vi "Main.vi"(11 "Module Admin":refnum<class "Delacor_lib_QMH_Module Admin.lvclass">) -> ()   [LabVIEW 2019, in "Rotation Stage.lvlib"]
doc: "This template is based off of the Queued Message Handler design pattern and the Queued Message Handler project template that ships with LabVIEW.\n\nThe main difference is that the queue is private to this module and communication between modules is performed via Broadcast and Request events.\n\nRequest events are wrapped in public API methods and are handled in the Event Handling Loop (EHL) of this VI. Any module can register for Broadcast events sent by this module. The EHL generates messages based on user interface actions.\n\nThe Message Handling Loop (MHL) processes messages generated by the EHL, or by other messages. The messages are string values, so new messages can be added easily to the Message Cases case structure in the MHL. Each message cluster can also provide an optional value for Message Data, which is a variant that can be converted to whatever message-specific data is required.\n_____\nBased on Delacor QMH Project Template 5.0.0.82."
uses:
  Rotation Stage.lvlib
  <vilib>/Delacor/Delacor QMH/Libraries/Module Admin_class/Delacor_lib_QMH_Module Admin.lvclass
  Module Data--cluster.ctl
  Stop Argument--cluster.ctl
  <vilib>/Delacor/Delacor QMH/Libraries/Message Queue_class/Delacor_lib_QMH_Message Queue.lvclass/Delacor_lib_QMH_Message Queue.ctl
  <vilib>/Delacor/Delacor QMH/Libraries/Module Admin_class/Delacor_lib_QMH_Module Admin.lvclass/Delacor_lib_QMH_Module Admin.ctl
  Get Position Argument--cluster.ctl
  Get Position (Reply Payload)--cluster.ctl
  Set Position Argument--cluster.ctl
  Get Module Data Argument--cluster.ctl
  Get Module Data (Reply Payload)--cluster.ctl
  <vilib>/Utility/miscctls.llb/LVPointTypeDef.ctl
  <vilib>/Delacor/Delacor QMH/Libraries/Message Queue_class/Delacor_lib_QMH_Enqueue Message (Single).vi
  <vilib>/Delacor/Delacor QMH/Libraries/Module Admin_class/Delacor_lib_QMH_Get External Launch.vi
  <vilib>/Utility/error.llb/Error Cluster From Error Code.vi
  <vilib>/ErrorRing/Error Ring.xnode
  <vilib>/Delacor/Delacor QMH/Libraries/Message Queue_class/Delacor_lib_QMH_Message Queue.lvclass
panel:
  in  "MG17Motor":refnum<k7>(container)
  out "error out":errorcluster
  out "Status":string
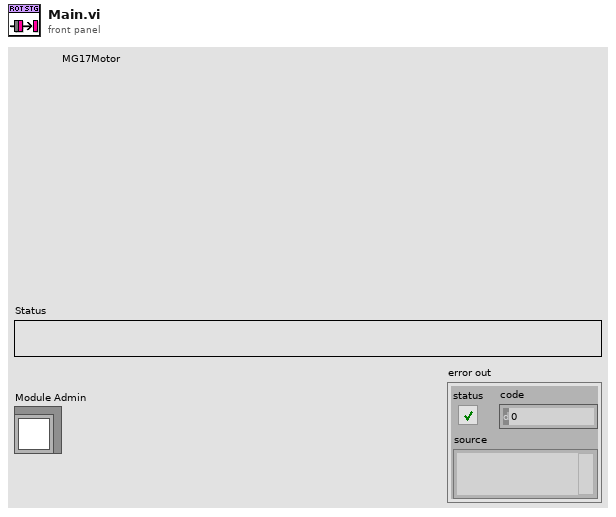
[diagram p1: front panel]
types:
  T1 = typedef "Rotation Stage.lvlib/Request Events--cluster.ctl" = cluster{"Stop Module":refnum<user-event>, "Show Panel":refnum<user-event>, "Hide Panel":refnum<user-event>, "Get Module Execution Status":refnum<user-event>, "Show Diagram":refnum<user-event>, "Get Position":refnum<user-event>, "Set Position":refnum<user-event>, "Get Module Data":refnum<user-event>}
  T2 = typedef "Rotation Stage.lvlib/Module Data--cluster.ctl" = cluster{"-Status":string, "-Reference":refnum<k7>, "Position":sgl}
  T3 = enum32{"invalid lock state", "Not Locked", "Locked (No Password)", "Password-protected"}
  T4 = typedef "Rotation Stage.lvlib/Stop Argument--cluster.ctl" = cluster{"Origin":string, "Exit via Stop Module Req?":bool, "Wait for Module to stop?":bool}
  T5 = typedef "Rotation Stage.lvlib/Get Position Argument--cluster.ctl" = cluster{"Wait Notifier":refnum<notifier>, "wait for reply":bool}
  T6 = typedef "Rotation Stage.lvlib/Set Position Argument--cluster.ctl" = cluster{"Position":sgl, "Wait":bool}
  T7 = typedef "Rotation Stage.lvlib/Get Module Data Argument--cluster.ctl" = cluster{"Wait Notifier":refnum<notifier>, "wait for reply":bool}
  T8 = typedef "LVPointTypeDef.ctl" = cluster{"Horizontal":i16, "Vertical":i16}
  T9 = enum32{"Invalid", "Standard", "Closed", "Hidden", "Minimized", "Maximized"}
  T10 = typedef "Rotation Stage.lvlib/Get Position (Reply Payload)--cluster.ctl" = cluster{"Position":dbl, "Get Position_error":errorcluster}
  T11 = typedef "Rotation Stage.lvlib/Get Module Data (Reply Payload)--cluster.ctl" = cluster{"Rotation Stage":T2, "Get Module Data_error":errorcluster}
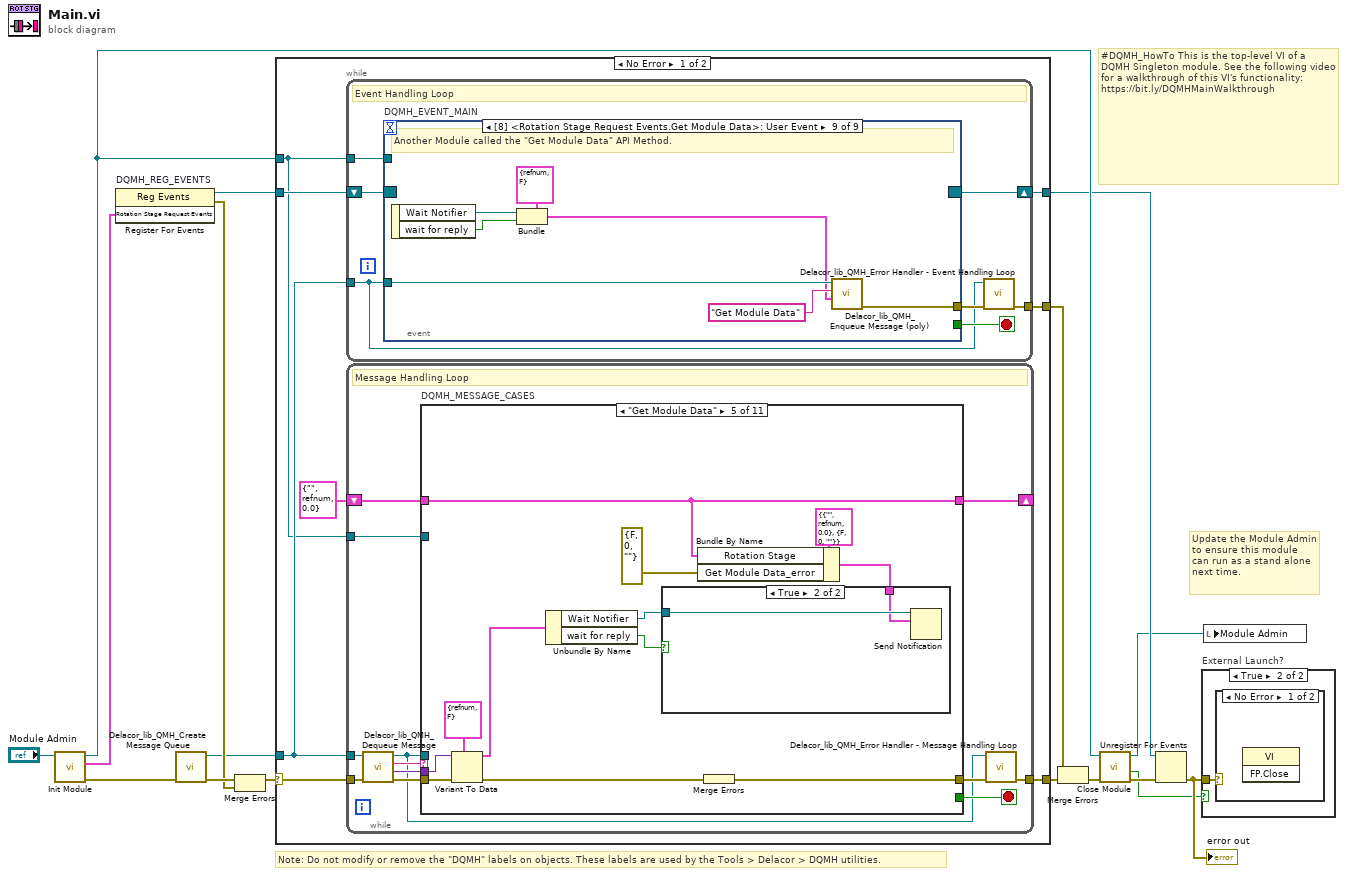
[diagram p0: block diagram]
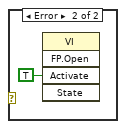
[diagram p3: hidden frame]
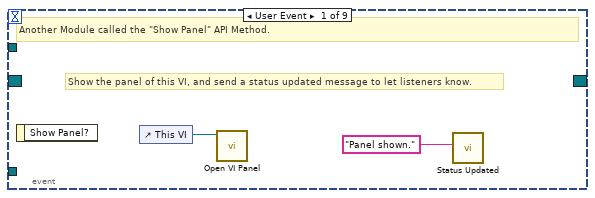
[diagram p4: hidden frame]
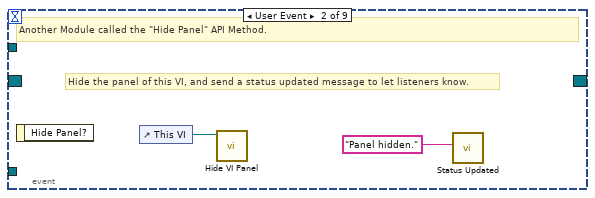
[diagram p5: hidden frame]
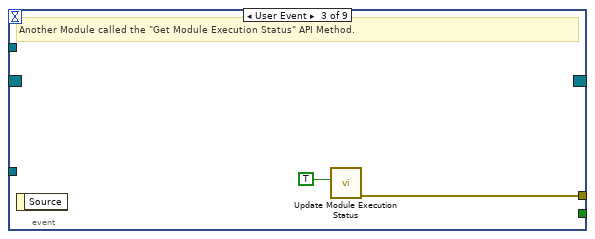
[diagram p6: hidden frame]
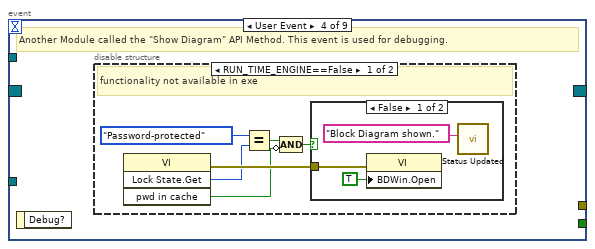
[diagram p7: hidden frame]
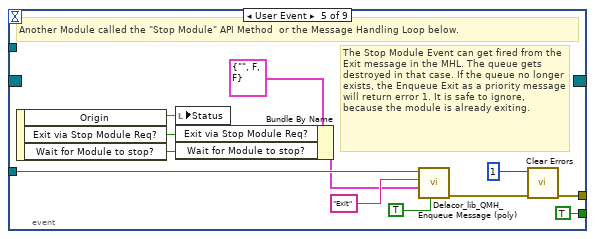
[diagram p10: hidden frame]
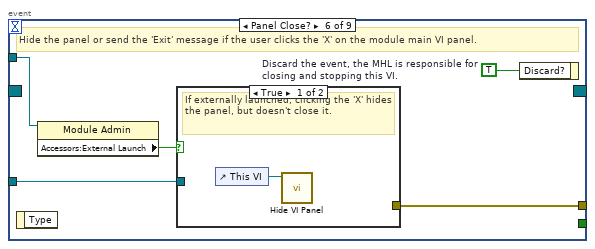
[diagram p11: hidden frame]
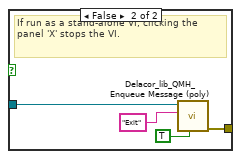
[diagram p12: hidden frame]
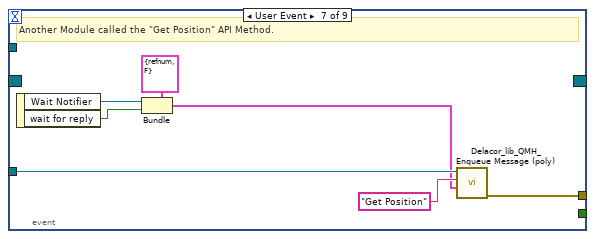
[diagram p13: hidden frame]
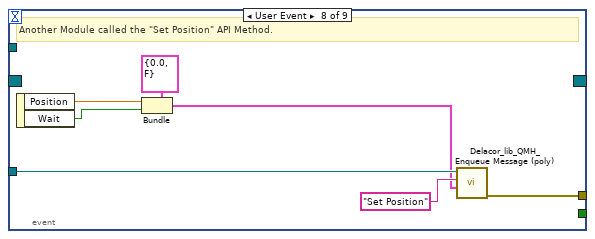
[diagram p14: hidden frame]
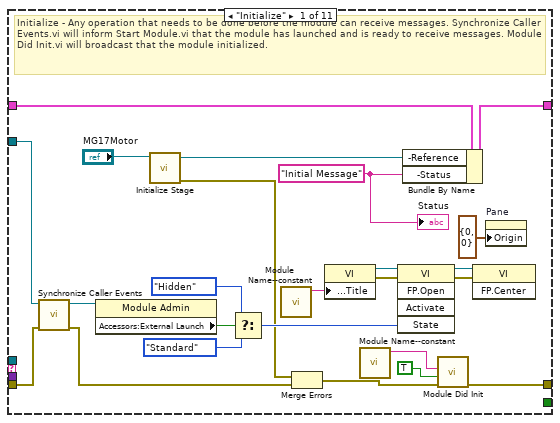
[diagram p15: hidden frame]
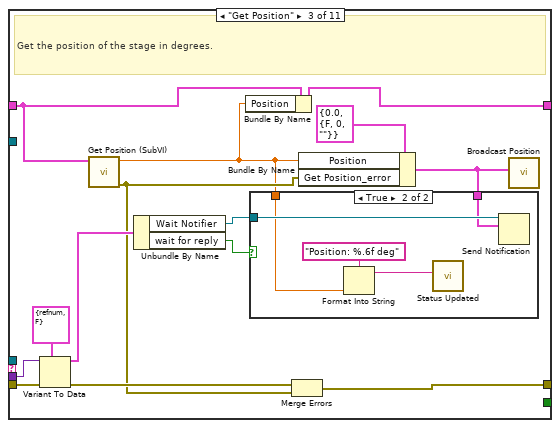
[diagram p17: hidden frame]
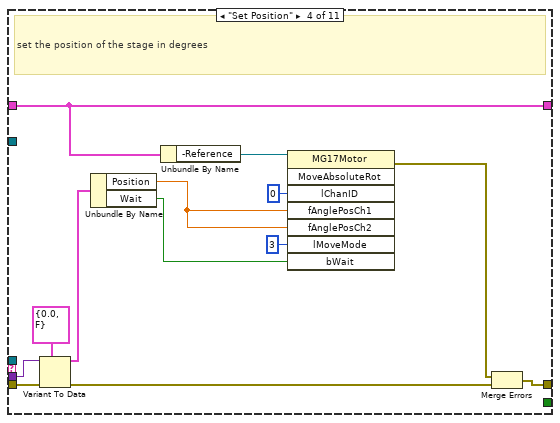
[diagram p19: hidden frame]
diagram:
  # "#DQMH_HowTo This is the top-level VI of a DQMH Singleton module. See the following video for a walkthrough of this VI's functionality: https://bit.ly/DQMHMainWalkthrough"
  # "Note: Do not modify or remove the \"DQMH\" labels on objects. These labels are used by the Tools > Delacor > DQMH utilities."
  # "Update the Module Admin to ensure this module can run as a stand alone next time."
  n1 = call "Init Module.vi"("Singleton Module Admin in"="Module Admin") -> ("error out"=w16:errorcluster, "Rotation Stage Request Events"=w5:T1, "Singleton Module Admin out"=w8:refnum<class "Delacor_lib_QMH_Module Admin.lvclass">)  [unwired: 8 in]
  n2 = register-events "DQMH_REG_EVENTS"(w5) -> (reference out=w6:refnum<event-registration>, error out=w9:errorcluster)  [unwired: 2 in]
  n3 = call <vilib>:"Delacor_lib_QMH_Create Message Queue.vi"("error in (no error)"=w16) -> ("error out"=w11:errorcluster, "Message Queue"=w4:refnum<class "Delacor_lib_QMH_Message Queue.lvclass">)  [unwired: 9 in]
  n4 = Merge Errors(w11, w9) -> (w10:errorcluster)
  n5 = case shown="No Error" w10 {
    selector: w10 -> [w23 w240]
    tunnel: [w25 w239] -> w17
    tunnel: [w22 w245] -> w7
    tunnel: w6 -> [w20 w245]
    tunnel: w4 -> [w19 w238]
    tunnel: [w24 _] -> w14
    tunnel: w8 -> [w18 w241]
    frame No Error {
      n6 = while {
        tunnel: w19 -> [w26]
        shift-right: [w29] -> w22
        shift-left: w20 -> [w30]
        tunnel: [w31] -> w24
        tunnel: w18 -> [w27]
        stop <- w28 stop-if-true
        # "Event Handling Loop"
        n7 = event "DQMH_EVENT_MAIN" shown="[8] <Rotation Stage Request Events.Get Module Data>: User Event" {
          selector: w30 -> [_ _ _ _ _ _ _ _ _]
          dyn-events: [_ _ _ _ _ _ _ _ _] -> w29
          timeout: _ -> [_ _ _ _ _ _ _ _ _]
          tunnel: [_ _ _ _ TRUE ("Discard?") _ _ _ _] -> w28
          tunnel: w26 -> [_ _ _ _ w55 w62 w76 w83 w90]
          tunnel: [_ _ w38 _ w58 w64 w70 w78 w84] -> w32
          tunnel: w27 -> [_ _ _ _ _ w61 _ _ _]
          event User Event {
            # "Show the panel of this VI, and send a status updated message to let listeners know."
            # "Another Module called the \"Show Panel\" API Method."
            n8 = event-data() -> ()  [unwired: 1 in, 1 out]
            n9 = control-ref of="This VI"() -> (w34:refnum<vi>)
            n10 = call "Open VI Panel.vi"("VI"=w34) -> ()  [unwired: 10 in, 1 out]
            n11 = call "Status Updated.vi"("Status"="Panel shown." ("format string")) -> ()  [unwired: 10 in, 1 out]
          }
          event User Event {
            # "Hide the panel of this VI, and send a status updated message to let listeners know."
            # "Another Module called the \"Hide Panel\" API Method."
            n12 = event-data() -> ()  [unwired: 1 in, 1 out]
            n13 = control-ref of="This VI"() -> (w36:refnum<vi>)
            n14 = call "Hide VI Panel.vi"("VI"=w36) -> ()  [unwired: 10 in, 1 out]
            n15 = call "Status Updated.vi"("Status"="Panel hidden." ("format string")) -> ()  [unwired: 10 in, 1 out]
          }
          event User Event {
            # "Another Module called the \"Get Module Execution Status\" API Method."
            n16 = event-data() -> ()  [unwired: 1 in, 1 out]
            n17 = call "Update Module Execution Status.vi"("Running?"=TRUE) -> ("error out"=w38:errorcluster)  [unwired: 10 in]
          }
          event User Event {
            # "Another Module called the \"Show Diagram\" API Method. This event is used for debugging."
            n18 = event-data() -> ()  [unwired: 1 in, 1 out]
            n19 = disable-structure shown="RUN_TIME_ENGINE==False" {
              frame condition #0 (active) {
                # "functionality not available in exe"
                n20 = invoke class="VI" method="Lock State.Get"() -> (error out=w44:errorcluster, "Get Lock State"=w43:T3, "pwd in cache"=w40:bool)  [unwired: 4 in, 1 out]
                n21 = Equal?(x=T3."Password-protected", y=w43) -> (x = y?=w41:bool)
                n22 = Compound Arithmetic op=AND(w41, invert w40) -> (w39:bool)
                n23 = case shown="False" w39 {
                  tunnel: w44 -> [w47 _]
                  frame False {
                    n24 = property class="VI"(error in=w47, "BDWin.Open"=TRUE ("Block Diagram Window:Open")) -> ()  [unwired: 1 in, 2 out]
                    n25 = call "Status Updated.vi"("Status"="Block Diagram shown." ("format string")) -> ()  [unwired: 10 in, 1 out]
                  }
                  frame True {
                    # "Password-protected VI, and the password is not in the cache. Do not show the diagram."
                  }
                }
              }
              frame condition #1 {
              }
            }
          }
          event User Event {
            # "The Stop Module Event can get fired from the Exit message in the MHL. The queue gets destroyed in that case. If the queue no longer exists, the Enqueue Exit as a priority message will return error 1. It is safe to ignore, because the module is already exiting."
            # "Another Module called the \"Stop Module\" API Method  or the Message Handling Loop below."
            n26 = event-data() -> ("Origin"=w54:string, "Exit via Stop Module Req?"=w50:bool, "Wait for Module to stop?"=w49:bool)  [unwired: 1 in]
            n27 = local write "Status"(w54) -> ()
            n28 = Bundle By Name(cluster=T4 {"Origin"="", "Exit via Stop Module Req?"=FALSE, "Wait for Module to stop?"=FALSE} ("Stop Argument"), "Exit via Stop Module Req?"=w50, "Wait for Module to stop?"=w49) -> (w48:T4)
            n29 = call-poly <vilib>:"Delacor_lib_QMH_Enqueue Message (poly).vi"("Priority Message? (F)"=TRUE, "Message Data"=w48, "Message"="Exit", "Message Queue in"=w55) -> ("error out"=w59:errorcluster)  [unwired: 6 in, 1 out]
            n30 = call <vilib>:"Clear Errors.vi"("error in (no error)"=w59, "specific error code to clear (0: all)"=1) -> ("error out"=w58:errorcluster)  [unwired: 4 in, 1 out]
          }
          event Panel Close? {
            w63 = TRUE  # Discard the event, the MHL is responsible for closing and stopping this VI.
            # "Hide the panel or send the 'Exit' message if the user clicks the 'X' on the module main VI panel."
            n31 = event-data() -> ()  [unwired: 1 in, 1 out]
            n32 = property class="Module Admin"(reference=w61) -> ("Accessors:External Launch"=w60:bool)  [unwired: 1 in, 2 out]
            n33 = case shown="True" w60 {
              tunnel: w62 -> [_ w68]
              tunnel: [_ w69] -> w64
              frame True {
                # "If externally launched, clicking the 'X' hides the panel, but doesn't close it."
                n34 = control-ref of="This VI"() -> (w65:refnum<vi>)
                n35 = call "Hide VI Panel.vi"("VI"=w65) -> ()  [unwired: 10 in, 1 out]
              }
              frame False {
                # "If run as a stand-alone VI, clicking the panel 'X' stops the VI."
                n36 = call-poly <vilib>:"Delacor_lib_QMH_Enqueue Message (poly).vi"("Priority Message? (F)"=TRUE, "Message"="Exit", "Message Queue in"=w68) -> ("error out"=w69:errorcluster)  [unwired: 7 in, 1 out]
              }
            }
            n37 = event-data("Discard?"=w63) -> ()  [unwired: 1 in, 1 out]
          }
          event User Event {
            # "Another Module called the \"Get Position\" API Method."
            n38 = event-data() -> ("Wait Notifier"=w72:refnum<notifier>, "wait for reply"=w71:bool)  [unwired: 1 in]
            n39 = Bundle(cluster=T5 {"Wait Notifier"=refnum, "wait for reply"=FALSE} ("Get Position Argument"), "Wait Notifier"=w72, "wait for reply"=w71) -> (w73:T5)
            n40 = call-poly <vilib>:"Delacor_lib_QMH_Enqueue Message (poly).vi"("Message Data"=w73, "Message"="Get Position", "Message Queue in"=w76) -> ("error out"=w70:errorcluster)  [unwired: 7 in, 1 out]
          }
          event User Event {
            # "Another Module called the \"Set Position\" API Method."
            n41 = event-data() -> ("Position"=w79:sgl, "Wait"=w77:bool)  [unwired: 1 in]
            n42 = Bundle(cluster=T6 {"Position"=0.0, "Wait"=FALSE} ("Set Position Argument"), "Position"=w79, "Wait"=w77) -> (w80:T6)
            n43 = call-poly <vilib>:"Delacor_lib_QMH_Enqueue Message (poly).vi"("Message Data"=w80, "Message"="Set Position", "Message Queue in"=w83) -> ("error out"=w78:errorcluster)  [unwired: 7 in, 1 out]
          }
          event User Event {
            # "Another Module called the \"Get Module Data\" API Method."
            n44 = event-data() -> ("Wait Notifier"=w86:refnum<notifier>, "wait for reply"=w85:bool)  [unwired: 1 in]
            n45 = Bundle(cluster=T7 {"Wait Notifier"=refnum, "wait for reply"=FALSE} ("Get Module Data Argument"), "Wait Notifier"=w86, "wait for reply"=w85) -> (w87:T7)
            n46 = call-poly <vilib>:"Delacor_lib_QMH_Enqueue Message (poly).vi"("Message Data"=w87, "Message"="Get Module Data", "Message Queue in"=w90) -> ("error out"=w84:errorcluster)  [unwired: 7 in, 1 out]
          }
        }
        n47 = call-dynamic "Delacor_lib_QMH_Error Handler - Event Handling Loop.vi"("error in (no error)"=w32, "Message Queue in"=w26) -> ("dup error in"=w31:errorcluster)  [unwired: 8 in, 1 out]
      }
      n48 = while {
        tunnel: w19 -> [w93]
        shift-right: [w97] -> _
        shift-left: T2 {"-Status"="", "-Reference"=refnum, "Position"=0.0} ("Data Cluster") -> [w98]
        tunnel: w23 -> [w101]
        tunnel: [w99] -> w25
        tunnel: w18 -> [w91]
        stop <- w96 stop-if-true
        # "Message Handling Loop"
        n49 = call-dynamic "Delacor_lib_QMH_Dequeue Message.vi"("error in (no error)"=w101, "Message Queue in"=w93) -> ("error out"=w100:errorcluster, "Message Data"=w94:variant, "Message"=w95:string, "Message Queue out"=w92:refnum<class "Delacor_lib_QMH_Message Queue.lvclass">)  [unwired: 6 in]
        n50 = case "DQMH_MESSAGE_CASES" shown="\"Get Module Data\"" w95 {
          selector: w95 -> [_ _ _ _ _ _ _ _ _ _ w225]
          tunnel: w92 -> [_ _ _ _ _ _ _ _ w195 w217 _]
          tunnel: w100 -> [w124 w128 w142 w160 w172 w177 w179 w184 w202 w223 w227]
          tunnel: [w122 w128 w133 w151 w163 w176 w179 w183 w198 w220 w228] -> w102
          tunnel: w98 -> [w113 w127 w132 w155 w162 w175 w178 w181 w197 w209 w226]
          tunnel: [w112 w127 w130 w155 w162 w175 w178 w181 w197 w209 w226] -> w97
          tunnel: [_ _ _ _ _ _ _ _ _ w216 _] -> w96
          tunnel: w94 -> [_ _ w140 w158 w170 _ _ _ w196 w215 _]
          tunnel: w91 -> [w114 _ _ _ _ _ _ _ w194 w210 _]
          frame "Initialize" {
            w107 = "Initial Message" ("Initial Message")
            # "Initialize - Any operation that needs to be done before the module can receive messages. Synchronize Caller Events.vi will inform Start Module.vi that the module has launched and is ready to receive messages. Module Did Init.vi will broadcast that the module initialized."
            n51 = call "Synchronize Caller Events.vi"("error in (no error)"=w124, "Singleton Module Admin in"=w114) -> ("error out"=w123:errorcluster, "Singleton Module Admin out"=w109:refnum<class "Delacor_lib_QMH_Module Admin.lvclass">)  [unwired: 8 in]
            n52 = property class="Module Admin"(reference=w109) -> ("Accessors:External Launch"=w118:bool)  [unwired: 1 in, 2 out]
            n53 = call "Initialize Stage.vi"("Automation Refnum in"="MG17Motor") -> ("error out"=w103:errorcluster, "reference out"=w105:refnum<k7>)  [unwired: 9 in]
            n54 = Select(t=T9."Hidden" ("State"), s=w118, f=T9."Standard" ("State")) -> (s? t:f=w115:T9)
            n55 = call "Module Name--constant.vi"() -> ("Module Name"=w121:string)  [unwired: 11 in]
            n56 = Merge Errors(w103, w123) -> (w104:errorcluster)
            n57 = property class="VI"("Front Panel.Title"=w121) -> (reference out=w120:refnum<vi>, error out=w126:errorcluster)  [unwired: 2 in]
            n58 = call "Module Name--constant.vi"() -> ("Module Name"=w110:string)  [unwired: 11 in]
            n59 = invoke class="VI" method="FP.Open"(reference=w120, error in=w126, "State"=w115) -> (reference out=w119:refnum<vi>, error out=w125:errorcluster)  [unwired: 2 in, 3 out]
            n60 = Bundle By Name(cluster=w113, "-Reference"=w105, "-Status"=w107) -> (w112:T2)
            n61 = call "Module Did Init.vi"("error in (no error)"=w104, "Initialized?"=TRUE, "Origin"=w110) -> ("error out"=w122:errorcluster)  [unwired: 8 in]
            n62 = invoke class="VI" method="FP.Center"(reference=w119, error in=w125) -> ()  [unwired: 1 in, 3 out]
            n63 = property on="Pane" class="Pane"("Origin"=T8 {"Horizontal"=0, "Vertical"=0}) -> ()  [unwired: 2 in, 2 out]
            "Status" <- w107
          }
          frame "--- Module Specific ---" {
            # "Separator -- The following cases handle messages specific to this Module."
          }
          frame "Get Position" {
            # "Get the position of the stage in degrees."
            n64 = Variant To Data(error in=w142, type=T5 {"Wait Notifier"=refnum, "wait for reply"=FALSE} ("Get Position Argument"), Variant=w140) -> (data=w138:T5, error out=w141:errorcluster)
            n65 = call "Get Position (SubVI).vi"("Data Cluster"=w132) -> ("error out"=w131:errorcluster, "pfPosition"=w129:sgl)  [unwired: 9 in]
            n66 = Unbundle By Name(w138) -> ("Wait Notifier"=w137:refnum<notifier>, "wait for reply"=w136:bool)
            n67 = Bundle By Name(cluster=w132, "Position"=w129) -> (w130:T2)
            n68 = Merge Errors(w141, w131) -> (w133:errorcluster)
            n69 = Bundle By Name(cluster=T10 {"Position"=0.0, "Get Position_error"={"status"=FALSE, "code"=0, "source"=""}} ("Get Position (Reply Payload)"), "Position"=w129, "Get Position_error"=w131) -> (w135:T10)
            n70 = case shown="True" w136 {
              tunnel: w137 -> [_ w147]
              tunnel: w135 -> [_ w146]
              tunnel: w129 -> [_ w144]
              frame False {
              }
              frame True {
                n71 = Format Into String(format string="Position: %.6f deg", w144) -> (resulting string=w143:string)  [unwired: 2 in, 1 out]
                n72 = call "Status Updated.vi"("Status"=w143) -> ()  [unwired: 10 in, 1 out]
                n73 = Send Notification(notification=w146, notifier=w147) -> ()  [unwired: 1 in, 2 out]
              }
            }
            n74 = call "Broadcast Position.vi"("Reply Payload"=w135) -> ()  [unwired: 10 in, 1 out]
          }
          frame "Set Position" {
            # "set the position of the stage in degrees"
            n75 = Variant To Data(error in=w160, type=T6 {"Position"=0.0, "Wait"=FALSE} ("Set Position Argument"), Variant=w158) -> (data=w156:T6, error out=w159:errorcluster)
            n76 = Unbundle By Name(w156) -> ("Position"=w149:sgl, "Wait"=w148:bool)
            n77 = Unbundle By Name(w155) -> ("-Reference"=w154:refnum<k7>)
            n78 = invoke class="MG17Motor" method="MoveAbsoluteRot"(reference=w154, "lChanID"=0, "fAnglePosCh1"=w149, "fAnglePosCh2"=w149, "lMoveMode"=3, "bWait"=w148) -> (error out=w150:errorcluster)  [unwired: 2 in, 7 out]
            n79 = Merge Errors(w150, w159) -> (w151:errorcluster)
          }
          frame "Get Module Data" {
            n80 = Variant To Data(error in=w172, type=T7 {"Wait Notifier"=refnum, "wait for reply"=FALSE} ("Get Module Data Argument"), Variant=w170) -> (data=w168:T7, error out=w171:errorcluster)
            n81 = Unbundle By Name(w168) -> ("Wait Notifier"=w167:refnum<notifier>, "wait for reply"=w166:bool)
            n82 = Bundle By Name(cluster=T11 {"Rotation Stage"={"-Status"="", "-Reference"=refnum, "Position"=0.0}, "Get Module Data_error"={"status"=FALSE, "code"=0, "source"=""}} ("Get Module Data (Reply Payload)"), "Rotation Stage"=w162, "Get Module Data_error"=errorcluster {"status"=FALSE, "code"=0, "source"=""}) -> (w165:T11)
            n83 = case shown="True" w166 {
              tunnel: w167 -> [_ w174]
              tunnel: w165 -> [_ w173]
              frame False {
              }
              frame True {
                n84 = Send Notification(notification=w173, notifier=w174) -> ()  [unwired: 1 in, 2 out]
              }
            }
            n85 = Merge Errors(w171) -> (w163:errorcluster)
          }
          frame "---Copy This Frame---" {
            # "Duplicate this frame when creating new messages.  Change this comment in the duplicated frame to describe this message."
            n86 = Merge Errors(w177) -> (w176:errorcluster)
          }
          frame "--- Exit and Error Handling---" {
            # "Separator - The following cases handle errors and exit messages."
          }
          frame "Simulate MHL Error" {
            # "#DQMH_HowTo The 'Simulate MHL Error' button  illustrates how the MHL handles errors. This event is instructional in nature and can be removed."
            # "Simulate an error occurring at the MHL"
            n87 = call "Module Name--constant.vi"() -> ("Module Name"=w180:string)  [unwired: 11 in]
            n88 = xnode "Error Ring"("parameter 0"=w180) -> ("error out"=w182:errorcluster)
            n89 = Merge Errors(w184, w182) -> (w183:errorcluster)
          }
          frame "Error" {
            # "#CodeRecommended - If you ever change the name of this \"Error\" message, you'll need to update the name in the Check Loop Error.vi as well."
            # "#CodeRecommended - If the module is running in standalone mode (External Launch = FALSE), this code will pop up an error dialog and call the 'Exit' message if an error occurs. Add more fine-grained error handling here."
            # "Error - Check the error message data and respond accordingly. This message is sent by the \"Error Handler\" VIs at the end of each loop in this application."
            n90 = property class="Module Admin"(reference=w194) -> ("Accessors:External Launch"=w193:bool)  [unwired: 1 in, 2 out]
            n91 = Variant To Data(error in=w202, type=errorcluster {"status"=FALSE, "code"=0, "source"=""} ("error constant"), Variant=w196) -> (data=w203:errorcluster, error out=w200:errorcluster)
            n92 = call "Module Name--constant.vi"() -> ("Module Name"=w192:string)  [unwired: 11 in]
            n93 = call "Error Reported.vi"("Additional Information"=w192, "Error"=w203) -> ()  [unwired: 9 in, 1 out]
            n94 = case shown="False" w193 {
              tunnel: [w208 _] -> w199
              tunnel: w195 -> [w206 _]
              tunnel: w203 -> [w207 _]
              frame False {
                # "If the module is running standalone, then pop up an error dialog and call the \"Exit\" message."
                n95 = call <vilib>:"Simple Error Handler.vi"("error in (no error)"=w207) -> ()  [unwired: 4 in, 5 out]
                n96 = call-poly <vilib>:"Delacor_lib_QMH_Enqueue Message (poly).vi"("Priority Message? (F)"=TRUE, "Message"="Exit", "Message Queue in"=w206) -> ("error out"=w208:errorcluster)  [unwired: 7 in, 1 out]
              }
              frame True {
                # "If the module was launched externally, calling the Error Reported broadcast VI is the only action performed by the \"Error\" message. The module's caller can then process the error appropriately."
              }
            }
            n97 = Merge Errors(w200, w199) -> (w198:errorcluster)
            n98 = local write "error out"(w198) -> ()
          }
          frame "Exit" {
            w214 = 91  # 91: not all Exit messages will have an argument
            w216 = TRUE  # Stop the VI
            # "Release the message queue reference"
            # "Exit - Exit the application."
            n99 = Variant To Data(error in=w223, type=T4 {"Origin"="", "Exit via Stop Module Req?"=FALSE, "Wait for Module to stop?"=FALSE} ("Stop Argument"), Variant=w215) -> (data=w212:T4, error out=w219:errorcluster)
            n100 = call <vilib>:"Clear Errors.vi"("error in (no error)"=w219, "specific error code to clear (0: all)"=w214) -> ("error out"=w222:errorcluster)  [unwired: 4 in, 1 out]
            n101 = call "Stop Control.vi"("Data Cluster"=w209) -> ()  [unwired: 11 in]
            n102 = control-ref of="This VI"() -> (w211:refnum<vi>)
            n103 = call-dynamic "Delacor_lib_QMH_Release Message Queue.vi"("error in (no error)"=w222, "Message Queue"=w217) -> ("error out"=w221:errorcluster)  [unwired: 9 in]
            n104 = call "Handle Exit.vi"("Stop Argument"=w212, "Admin in"=w210, "VI reference"=w211) -> ("error out"=w218:errorcluster)  [unwired: 7 in, 1 out]
            n105 = Merge Errors(w221, w218) -> (w220:errorcluster)
          }
          frame Default {
            # "'Default' case only runs if there is a message that isn't defined in any of the other cases.  Output a programming error."
            n106 = call "Module Name--constant.vi"() -> ("Module Name"=w224:string)  [unwired: 11 in]
            n107 = xnode "Error Ring"("parameter 0"=w225, "parameter 1"=w224) -> ("error out"=w229:errorcluster)
            n108 = Merge Errors(w227, w229) -> (w228:errorcluster)
          }
        }
        n109 = call-dynamic "Delacor_lib_QMH_Error Handler - Message Handling Loop.vi"("error in (no error)"=w102, "Message Queue in"=w92) -> ("dup error in"=w99:errorcluster)  [unwired: 8 in, 1 out]
      }
    }
    frame Error {
      # "Synchronize Caller Events.vi will inform Start Module.vi that the module has launched and will let the code calling Start Module.vi register for broadcasts and would permit the caller receive the broadcast that an error occurred at launch time."
      n110 = call-dynamic "Delacor_lib_QMH_Release Message Queue.vi"("error in (no error)"=w240, "Message Queue"=w238) -> ("error out"=w239:errorcluster)  [unwired: 9 in]
      n111 = call "Synchronize Caller Events.vi"("Singleton Module Admin in"=w241) -> ("error out"=w246:errorcluster)  [unwired: 9 in, 1 out]
      n112 = call "Module Name--constant.vi"() -> ("Module Name"=w244:string)  [unwired: 11 in]
      n113 = Format Into String(format string="An error occurred during initialization. %s is no longer running.", w244) -> (resulting string=w242:string)  [unwired: 2 in, 1 out]
      n114 = Merge Errors(w239, w246) -> (w247:errorcluster)
      n115 = call "Error Reported.vi"("Additional Information"=w242, "Error"=w247) -> ()  [unwired: 9 in, 1 out]
    }
  }
  n116 = Merge Errors(w14, w17) -> (w13:errorcluster)
  n117 = call "Close Module.vi"("error in (no error)"=w13, "Module Admin in"=w8) -> ("error out"=w15:errorcluster, "External Launch"=w1:bool, "Module Admin out"=w2:refnum<class "Delacor_lib_QMH_Module Admin.lvclass">)  [unwired: 7 in]
  n118 = Unregister For Events(event registration refnum=w7, error in=w15) -> (error out=w12:errorcluster)
  "error out" <- w12
  n119 = case "External Launch?" shown="True" w1 {
    tunnel: w12 -> [_ w248]
    frame False {
    }
    frame True {
      n120 = case shown="No Error" w248 {
        frame No Error {
          n121 = invoke class="VI" method="FP.Close"() -> ()  [unwired: 3 in, 3 out]
        }
        frame Error {
          n122 = invoke class="VI" method="FP.Open"("Activate"=TRUE ("Activate?")) -> ()  [unwired: 4 in, 5 out]
        }
      }
    }
  }
  n123 = local write "Module Admin"(w2) -> ()
